vi "nism.digitalFilter.u8(modified).vi"(6 "filter value (us)":u16=2000, 11 "input signal":u8) -> (3 "output signal":u8)   [LabVIEW 2014]
doc: "Applies the user specified digital filter to the input signal or signals. Filter settings are specified using either the Axis Configuration dialog box or using the appropriate Axis property."
uses:
  <vilib>/Motion/MotorControl/NI_SoftMotion_MotorControlIP.lvlib
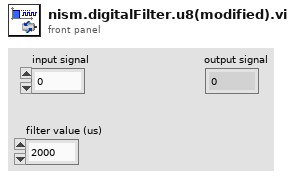
[diagram p1: front panel]
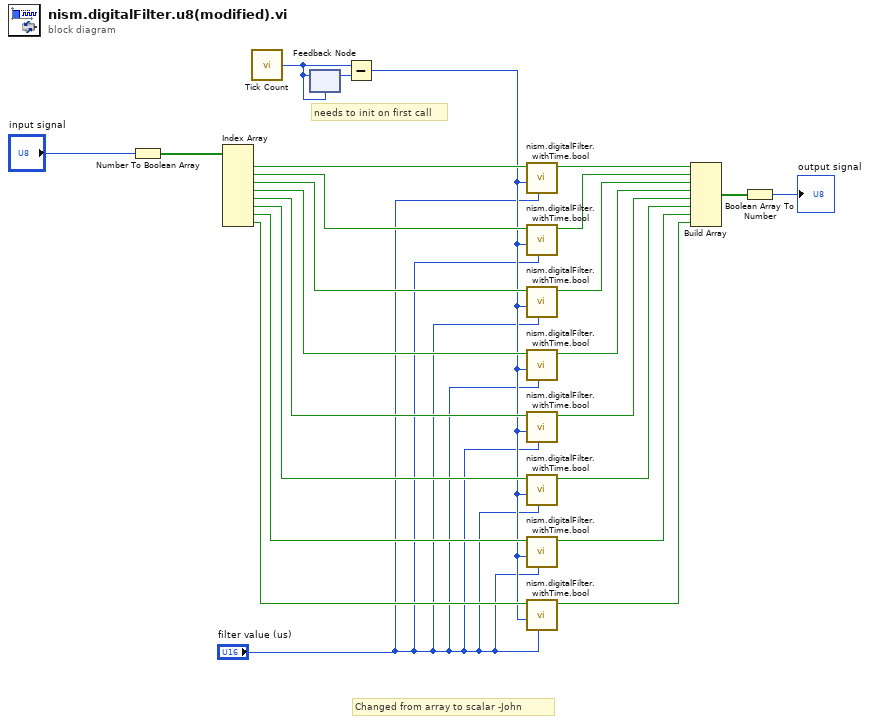
[diagram p0: block diagram]
diagram:
  # "Changed from array to scalar -John"
  # "needs to init on first call"
  n1 = Number To Boolean Array(number="input signal") -> (Boolean array=w23:bool[])
  n2 = Index Array(array=w23) -> (element #1=w22:bool, element #2=w15:bool, element #3=w16:bool, element #4=w17:bool, element #5=w18:bool, element #6=w19:bool, element #7=w20:bool, element #8=w21:bool)  [unwired: 8 in]
  n3 = call "Tick Count"() -> ("Tick Count(uSec)"=w3:u16)
  n4 = feedback #1(w3) -> (w4:u16)
  n5 = feedback-in #1(w3) -> ()
  n6 = Subtract(x=w3, y=w4) -> (x-y=w2:u16)
  n7 = call <vilib>:"nism.digitalFilter.withTime.bool.vi"("filter value"="filter value (us)", "delta time"=w2, "input signal"=w22) -> ("output signal"=w14:bool)  [unwired: 8 in]
  n8 = call <vilib>:"nism.digitalFilter.withTime.bool.vi"("filter value"="filter value (us)", "delta time"=w2, "input signal"=w15) -> ("output signal"=w7:bool)  [unwired: 8 in]
  n9 = call <vilib>:"nism.digitalFilter.withTime.bool.vi"("filter value"="filter value (us)", "delta time"=w2, "input signal"=w16) -> ("output signal"=w8:bool)  [unwired: 8 in]
  n10 = call <vilib>:"nism.digitalFilter.withTime.bool.vi"("filter value"="filter value (us)", "delta time"=w2, "input signal"=w17) -> ("output signal"=w9:bool)  [unwired: 8 in]
  n11 = call <vilib>:"nism.digitalFilter.withTime.bool.vi"("filter value"="filter value (us)", "delta time"=w2, "input signal"=w18) -> ("output signal"=w10:bool)  [unwired: 8 in]
  n12 = call <vilib>:"nism.digitalFilter.withTime.bool.vi"("filter value"="filter value (us)", "delta time"=w2, "input signal"=w19) -> ("output signal"=w11:bool)  [unwired: 8 in]
  n13 = call <vilib>:"nism.digitalFilter.withTime.bool.vi"("filter value"="filter value (us)", "delta time"=w2, "input signal"=w20) -> ("output signal"=w12:bool)  [unwired: 8 in]
  n14 = call <vilib>:"nism.digitalFilter.withTime.bool.vi"("filter value"="filter value (us)", "delta time"=w2, "input signal"=w21) -> ("output signal"=w13:bool)  [unwired: 8 in]
  n15 = Build Array(w14, w7, w8, w9, w10, w11, w12, w13) -> (w6:bool[])
  n16 = Boolean Array To Number(Boolean array=w6) -> (number=→"output signal":u8)
